vi "GetParameters.vi"() -> ()   [LabVIEW 2019]
panel:
  out "appended array 3":cluster{dbl, dbl}[][](array[cluster])
  out "MatrixPoint":cluster{dbl, dbl}[][](array[cluster])
  out "appended array":cluster{"X":dbl, "Y":dbl}[][](array[cluster])
  out "Particle Measurements (Real-World) (Particle Analysis 1)":dbl[][](array[numeric]) format="%.2f"
  out "Number of Particles (Particle Analysis 1)":i32
  out "CalImgOut":T1(plugin-control)
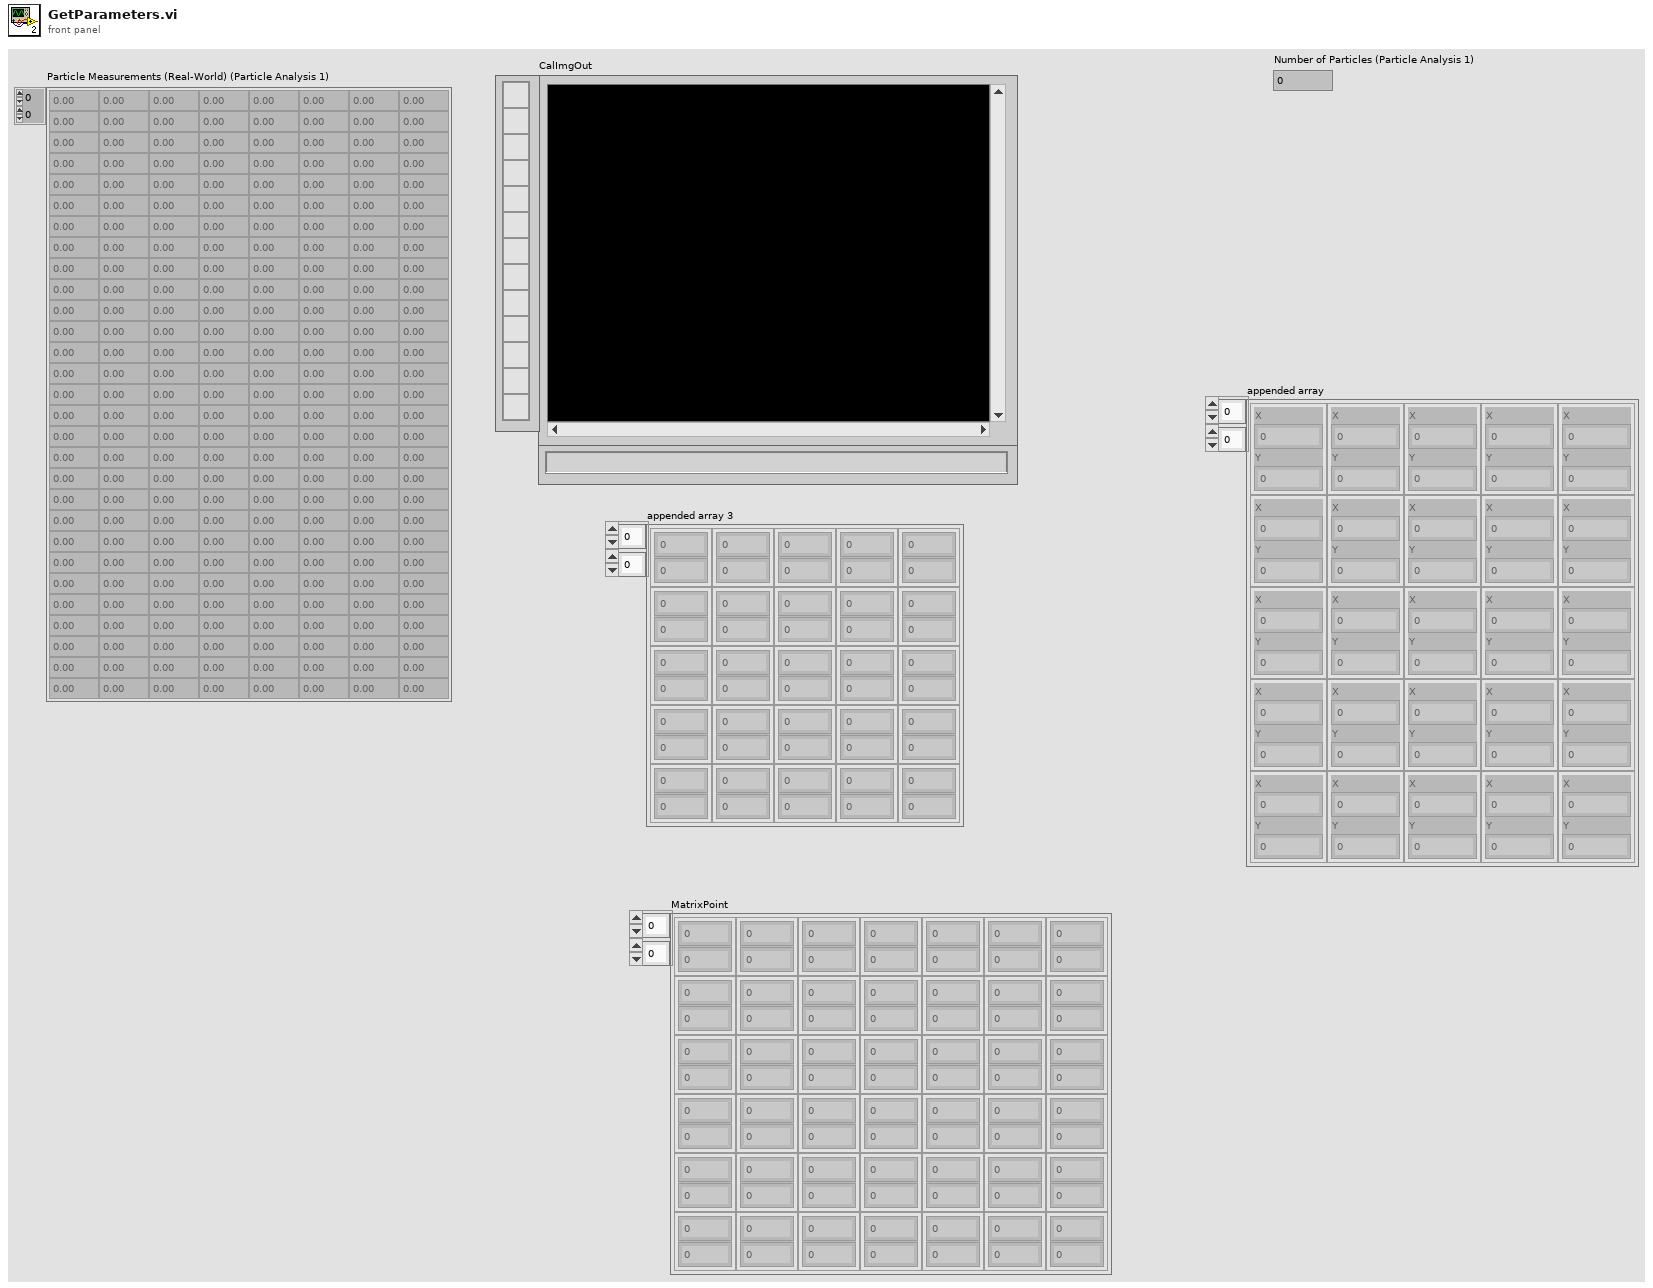
[diagram p1: front panel]
types:
  T1 = typedef "IMAQ Image.ctl" = refnum<image>
  T2 = typedef "Image Type" = u32
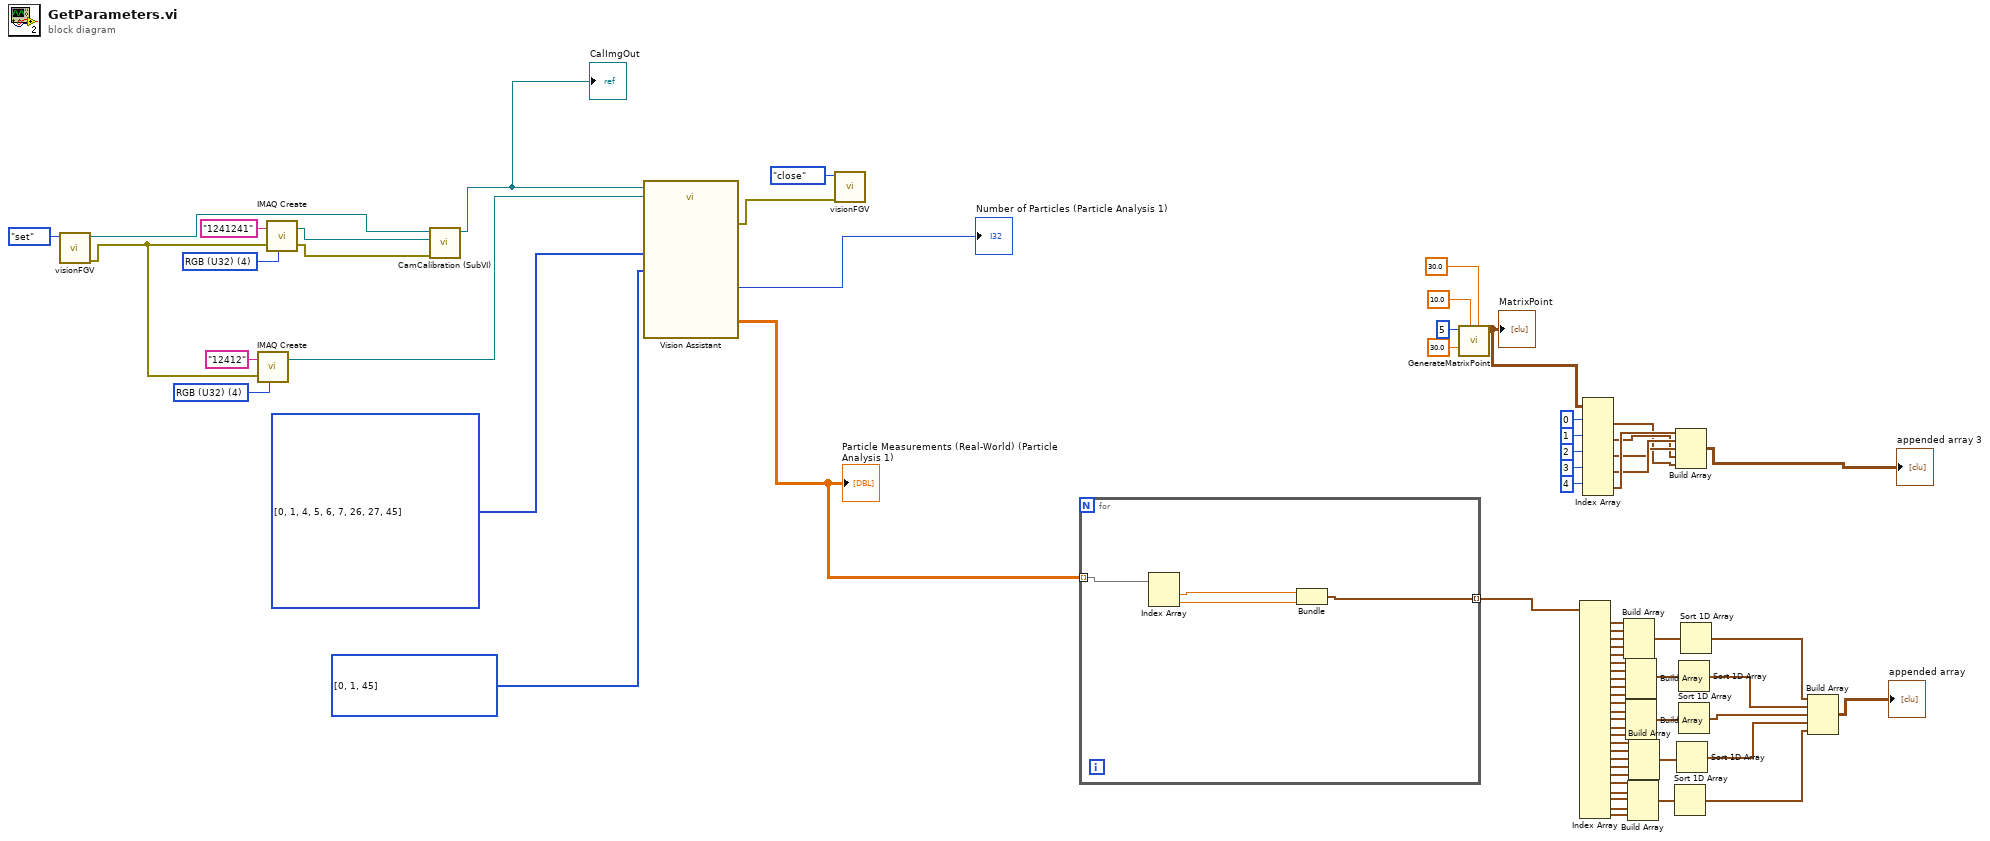
[diagram p0: block diagram]
diagram:
  w55 = i32[] [0, 1, 45] items=["Center of Mass X", "Center of Mass Y", "First Pixel X", "First Pixel Y", "Bounding Rect Left", "Bounding Rect Top", "Bounding Rect Right", "Bounding Rect Bottom", "Max Feret Diameter Start X", "Max Feret Diameter Start Y", "Max Feret Diameter End X", "Max Feret Diameter End Y", "Max Horiz. Segment Length Left", "Max Horiz. Segment Length Right", "Max Horiz. Segment Length Row", "-", "Bounding Rect Width", "Bounding Rect Height", "Bounding Rect Diagonal", "Perimeter", "Convex Hull Perimeter", "Holes' Perimeter", "Max Feret Diameter", "Equivalent Ellipse Major Axis", "Equivalent Ellipse Minor Axis", "Equivalent Ellipse Minor Axis (Feret)", "Equivalent Rect Long Side", "Equivalent Rect Short Side", "Equivalent Rect Diagonal", "Equivalent Rect Short Side (Feret)", "Average Horiz. Segment Length", "Average Vert. Segment Length", "Hydraulic Radius", "Waddel Disk Diameter", "-", "Area", "Holes' Area", "Particle & Holes' Area", "Convex Hull Area", "Image Area", "-", "Number of Holes", "Number of Horiz. Segments", "Number of Vert. Segments", "-", "Orientation", "Max Feret Diameter Orientation", "-", "% Area/Image Area", "% Area/(Particle & Holes' Area)", "Ratio of Equivalent Ellipse Axes", "Ratio of Equivalent Rect Sides", "-", "Elongation Factor", "Compactness Factor", "Heywood Circularity Factor", "Type Factor", "-", "Sum X", "Sum Y", "Sum XX", "Sum XY", "Sum YY", "Sum XXX", "Sum XXY", "Sum XYY", "Sum YYY", "-", "Moment of Inertia XX", "Moment of Inertia XY", "Moment of Inertia YY", "Moment of Inertia XXX", "Moment of Inertia XXY", "Moment of Inertia XYY", "Moment of Inertia YYY", "Norm. Moment of Inertia XX", "Norm. Moment of Inertia XY", "Norm. Moment of Inertia YY", "Norm. Moment of Inertia XXX", "Norm. Moment of Inertia XXY", "Norm. Moment of Inertia XYY", "Norm. Moment of Inertia YYY", "Hu Moment 1", "Hu Moment 2", "Hu Moment 3", "Hu Moment 4", "Hu Moment 5", "Hu Moment 6", "Hu Moment 7"] ("Real-World Measurements (Particle Analysis 1)")
  w56 = i32[] [0, 1, 4, 5, 6, 7, 26, 27, 45] items=["Center of Mass X", "Center of Mass Y", "First Pixel X", "First Pixel Y", "Bounding Rect Left", "Bounding Rect Top", "Bounding Rect Right", "Bounding Rect Bottom", "Max Feret Diameter Start X", "Max Feret Diameter Start Y", "Max Feret Diameter End X", "Max Feret Diameter End Y", "Max Horiz. Segment Length Left", "Max Horiz. Segment Length Right", "Max Horiz. Segment Length Row", "-", "Bounding Rect Width", "Bounding Rect Height", "Bounding Rect Diagonal", "Perimeter", "Convex Hull Perimeter", "Holes' Perimeter", "Max Feret Diameter", "Equivalent Ellipse Major Axis", "Equivalent Ellipse Minor Axis", "Equivalent Ellipse Minor Axis (Feret)", "Equivalent Rect Long Side", "Equivalent Rect Short Side", "Equivalent Rect Diagonal", "Equivalent Rect Short Side (Feret)", "Average Horiz. Segment Length", "Average Vert. Segment Length", "Hydraulic Radius", "Waddel Disk Diameter", "-", "Area", "Holes' Area", "Particle & Holes' Area", "Convex Hull Area", "Image Area", "-", "Number of Holes", "Number of Horiz. Segments", "Number of Vert. Segments", "-", "Orientation", "Max Feret Diameter Orientation", "-", "% Area/Image Area", "% Area/(Particle & Holes' Area)", "Ratio of Equivalent Ellipse Axes", "Ratio of Equivalent Rect Sides", "-", "Elongation Factor", "Compactness Factor", "Heywood Circularity Factor", "Type Factor", "-", "Sum X", "Sum Y", "Sum XX", "Sum XY", "Sum YY", "Sum XXX", "Sum XXY", "Sum XYY", "Sum YYY", "-", "Moment of Inertia XX", "Moment of Inertia XY", "Moment of Inertia YY", "Moment of Inertia XXX", "Moment of Inertia XXY", "Moment of Inertia XYY", "Moment of Inertia YYY", "Norm. Moment of Inertia XX", "Norm. Moment of Inertia XY", "Norm. Moment of Inertia YY", "Norm. Moment of Inertia XXX", "Norm. Moment of Inertia XXY", "Norm. Moment of Inertia XYY", "Norm. Moment of Inertia YYY", "Hu Moment 1", "Hu Moment 2", "Hu Moment 3", "Hu Moment 4", "Hu Moment 5", "Hu Moment 6", "Hu Moment 7"] ("Pixel Measurements (Particle Analysis 1)")
  w68 = T2 4 items=["Grayscale (U8)", "Grayscale (I16)", "Grayscale (SGL)", "Complex (CSG)", "RGB (U32)", "HSL (U32)", "RGB (U64)", "Grayscale (U16)"] ("Image Type")
  w69 = T2 4 items=["Grayscale (U8)", "Grayscale (I16)", "Grayscale (SGL)", "Complex (CSG)", "RGB (U32)", "HSL (U32)", "RGB (U64)", "Grayscale (U16)"] ("Image Type")
  n1 = call "visionFGV.vi"("Function"=enum16{"set", "read", "close"}."set") -> ("error out"=w63:errorcluster, "Image Out fgv"=w61:T1)  [unwired: 9 in]
  n2 = call "IMAQ Create"("Image Name"="12412", "Image Type"=w68, "error in (no error)"=w63) -> ("New Image"=w66:T1)  [unwired: 2 in, 1 out]
  n3 = call "IMAQ Create"("Image Name"="1241241", "Image Type"=w69, "error in (no error)"=w63) -> ("New Image"=w65:T1, "error out"=w62:errorcluster)  [unwired: 2 in]
  n4 = call "CamCalibration (SubVI).vi"("error in"=w62, "Image Dst"=w65, "Image In"=w61) -> ("Image Out"=w60:T1)  [unwired: 7 in, 1 out]
  "CalImgOut" <- w60
  n5 = call "Vision Assistant"("Image In"=w60, "Image Dst"=w66, "Pixel Measurements (Particle Analysis 1)"=w56, "Real-World Measurements (Particle Analysis 1)"=w55) -> ("Particle Measurements (Real-World) (Particle Analysis 1)"=w54:dbl[][], "Number of Particles (Particle Analysis 1)"=→"Number of Particles (Particle Analysis 1)":i32, "error out"=w59:errorcluster)  [unwired: 19 in, 2 out]
  "Particle Measurements (Real-World) (Particle Analysis 1)" <- w54
  n6 = call "visionFGV.vi"("Error In"=w59, "Function"=enum16{"set", "read", "close"}."close") -> ()  [unwired: 8 in, 2 out]
  n7 = for {
    tunnel: w54 -> [w74] mode=indexing
    tunnel: [w71] -> w14 mode=indexing
    n8 = Index Array(array=w74) -> (element #1=w73:dbl, element #2=w72:dbl)  [unwired: 2 in]
    n9 = Bundle("Numeric"=w73, "Numeric"=w72) -> (w71:cluster{"Numeric":dbl, "Numeric":dbl})  [unwired: 1 in]
  }
  n10 = call "GenerateMatrixPoint.vi"("YOffSet"=30.0, "XOffSet"=10.0, "Pitch"=30.0, "MatrixSize"=5) -> ("MatrixPoint"=w2:cluster{dbl, dbl}[][])  [unwired: 6 in, 1 out]
  "MatrixPoint" <- w2
  n11 = Index Array(array=w14) -> (element #1=w40:cluster{"Numeric":dbl, "Numeric":dbl}, element #2=w49:cluster{"Numeric":dbl, "Numeric":dbl}, element #3=w48:cluster{"Numeric":dbl, "Numeric":dbl}, element #4=w47:cluster{"Numeric":dbl, "Numeric":dbl}, element #5=w46:cluster{"Numeric":dbl, "Numeric":dbl}, element #6=w45:cluster{"Numeric":dbl, "Numeric":dbl}, element #7=w44:cluster{"Numeric":dbl, "Numeric":dbl}, element #8=w41:cluster{"Numeric":dbl, "Numeric":dbl}, element #9=w43:cluster{"Numeric":dbl, "Numeric":dbl}, element #10=w42:cluster{"Numeric":dbl, "Numeric":dbl}, element #11=w37:cluster{"Numeric":dbl, "Numeric":dbl}, element #12=w36:cluster{"Numeric":dbl, "Numeric":dbl}, element #13=w35:cluster{"Numeric":dbl, "Numeric":dbl}, element #14=w34:cluster{"Numeric":dbl, "Numeric":dbl}, element #15=w33:cluster{"Numeric":dbl, "Numeric":dbl}, element #16=w32:cluster{"Numeric":dbl, "Numeric":dbl}, element #17=w31:cluster{"Numeric":dbl, "Numeric":dbl}, element #18=w30:cluster{"Numeric":dbl, "Numeric":dbl}, element #19=w29:cluster{"Numeric":dbl, "Numeric":dbl}, element #20=w28:cluster{"Numeric":dbl, "Numeric":dbl}, element #21=w27:cluster{"Numeric":dbl, "Numeric":dbl}, element #22=w26:cluster{"Numeric":dbl, "Numeric":dbl}, element #23=w25:cluster{"Numeric":dbl, "Numeric":dbl}, element #24=w24:cluster{"Numeric":dbl, "Numeric":dbl}, element #25=w23:cluster{"Numeric":dbl, "Numeric":dbl})  [unwired: 25 in]
  n12 = Index Array(array=w2, index (row) #1=0 ("index (row)"), index (row) #2=1 ("index (row)"), index (row) #3=2 ("index (row)"), index (row) #4=3 ("index (row)"), index (row) #5=4 ("index (row)")) -> (element #1=w3:cluster{dbl, dbl}[], element #2=w4:cluster{dbl, dbl}[], element #3=w5:cluster{dbl, dbl}[], element #4=w6:cluster{dbl, dbl}[], element #5=w7:cluster{dbl, dbl}[])  [unwired: 5 in]
  n13 = Build Array(w40, w49, w48, w47, w46) -> (w39:cluster{"Numeric":dbl, "Numeric":dbl}[])
  n14 = Build Array(w45, w44, w41, w43, w42) -> (w38:cluster{"Numeric":dbl, "Numeric":dbl}[])
  n15 = Build Array(w37, w36, w35, w34, w33) -> (w20:cluster{"Numeric":dbl, "Numeric":dbl}[])
  n16 = Build Array(w27, w26, w25, w24, w23) -> (w22:cluster{"Numeric":dbl, "Numeric":dbl}[])
  n17 = Build Array(w32, w31, w30, w29, w28) -> (w21:cluster{"Numeric":dbl, "Numeric":dbl}[])
  n18 = Sort 1D Array(array=w22) -> (sorted array=w15:cluster{"Numeric":dbl, "Numeric":dbl}[])
  n19 = Build Array(w7, w6, w5, w4, w3) -> (→"appended array 3":cluster{dbl, dbl}[][])
  n20 = Sort 1D Array(array=w21) -> (sorted array=w16:cluster{"Numeric":dbl, "Numeric":dbl}[])
  n21 = Sort 1D Array(array=w38) -> (sorted array=w18:cluster{"Numeric":dbl, "Numeric":dbl}[])
  n22 = Sort 1D Array(array=w20) -> (sorted array=w17:cluster{"Numeric":dbl, "Numeric":dbl}[])
  n23 = Sort 1D Array(array=w39) -> (sorted array=w19:cluster{"Numeric":dbl, "Numeric":dbl}[])
  n24 = Build Array(w19, w18, w17, w16, w15) -> (→"appended array":cluster{"Numeric":dbl, "Numeric":dbl}[][])
